vi "Get Paths.vi"(7 "Extension(txt)":string="txt", 8 "error in":errorcluster, 10 "VI name":string) -> (0 "error out":errorcluster, 2 "recived path":path, 3 "approved path":path)   [LabVIEW 2020, in "Approval Tests.lvlib"]
doc: "Generates 2 absolute paths based on the name of the calling unit test.\n\nname_of_unit_test.approved\nname_of_unit_test.actual"
uses:
  Approval Tests.lvlib
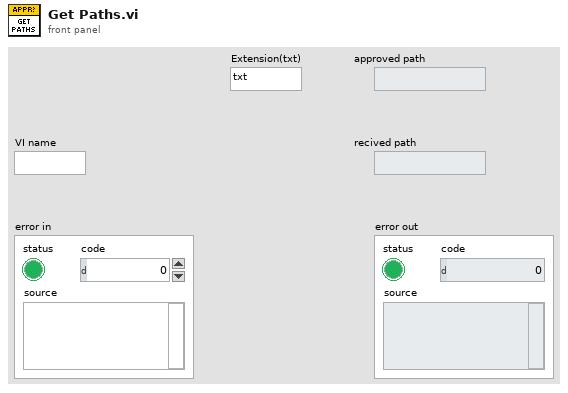
[diagram p1: front panel]
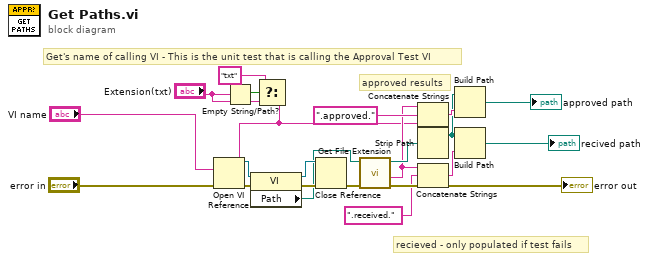
[diagram p0: block diagram]
diagram:
  # "recieved - only populated if test fails"
  # "approved results"
  # "Get's name of calling VI - This is the unit test that is calling the Approval Test VI"
  n1 = Open VI Reference(vi path="VI name", error in (no error)="error in") -> (vi reference=w14:refnum<vi>, error out=w18:errorcluster)  [unwired: 4 in]
  n2 = Empty String/Path?(string/path="Extension(txt)") -> (empty?=w4:bool)
  n3 = property on="Property Node" class="VI"(reference=w14, error in=w18) -> (reference out=w16:refnum<vi>, error out=w19:errorcluster, "Path"=w15:path)
  n4 = Select(t="txt", s=w4, f="Extension(txt)") -> (s? t:f=w2:string)
  n5 = Close Reference(reference=w16, error in (no error)=w19) -> (error out=w20:errorcluster)
  n6 = call <vilib>:"Get File Extension.vi"("error in (no error)"=w20, "file"=w15) -> ("error out"=→"error out":errorcluster, "filename without extension"=w6:string, "dup file"=w11:path)  [unwired: 5 in, 2 out]
  n7 = Concatenate Strings(w6, ".approved." ("string"), w2) -> (w13:string)
  n8 = Strip Path(path=w11) -> (stripped path=w8:path)  [unwired: 1 out]
  n9 = Concatenate Strings(w6, ".received." ("string"), w2) -> (w9:string)
  n10 = Build Path(base path=w8, name or relative path=w13) -> (appended path=→"approved path":path)
  n11 = Build Path(base path=w8, name or relative path=w9) -> (appended path=→"recived path":path)
